vi "_builtins_label_rename.vi"(8 "error in (no error)":errorcluster, 10 "Label":string, 11 "GObject in":refnum<vi>) -> (0 "error out":errorcluster, 2 "has label?":bool, 3 "GObject out":refnum<vi>)   [LabVIEW 2019, in "Script.lvlib"]
doc: "Renames the GObject label if exists and moves the label to the appropriate position.\n\nCreated by: Ryan Pacini"
uses:
  Script.lvlib
  _builtins_label_position.ctl
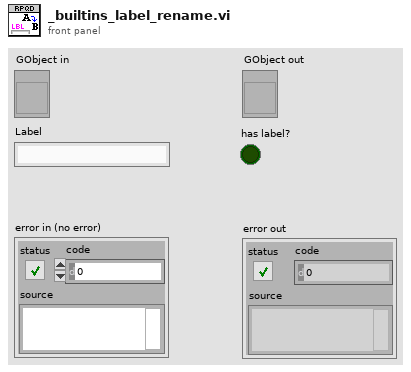
[diagram p1: front panel]
types:
  T1 = typedef "Script.lvlib/_builtins_label_position.ctl" = enum8{"Unchanged", "Top-left", "Top-middle", "Top-right", "Right-top", "Right-middle", "Right-bottom", "Bottom-right", "Bottom-middle", "Bottom-left", "Left-bottom", "Left-middle", "Left-top"}
  T2 = typedef "LVRectTypeDef.ctl" = cluster{"Left":i16, "Top":i16, "Right":i16, "Bottom":i16}
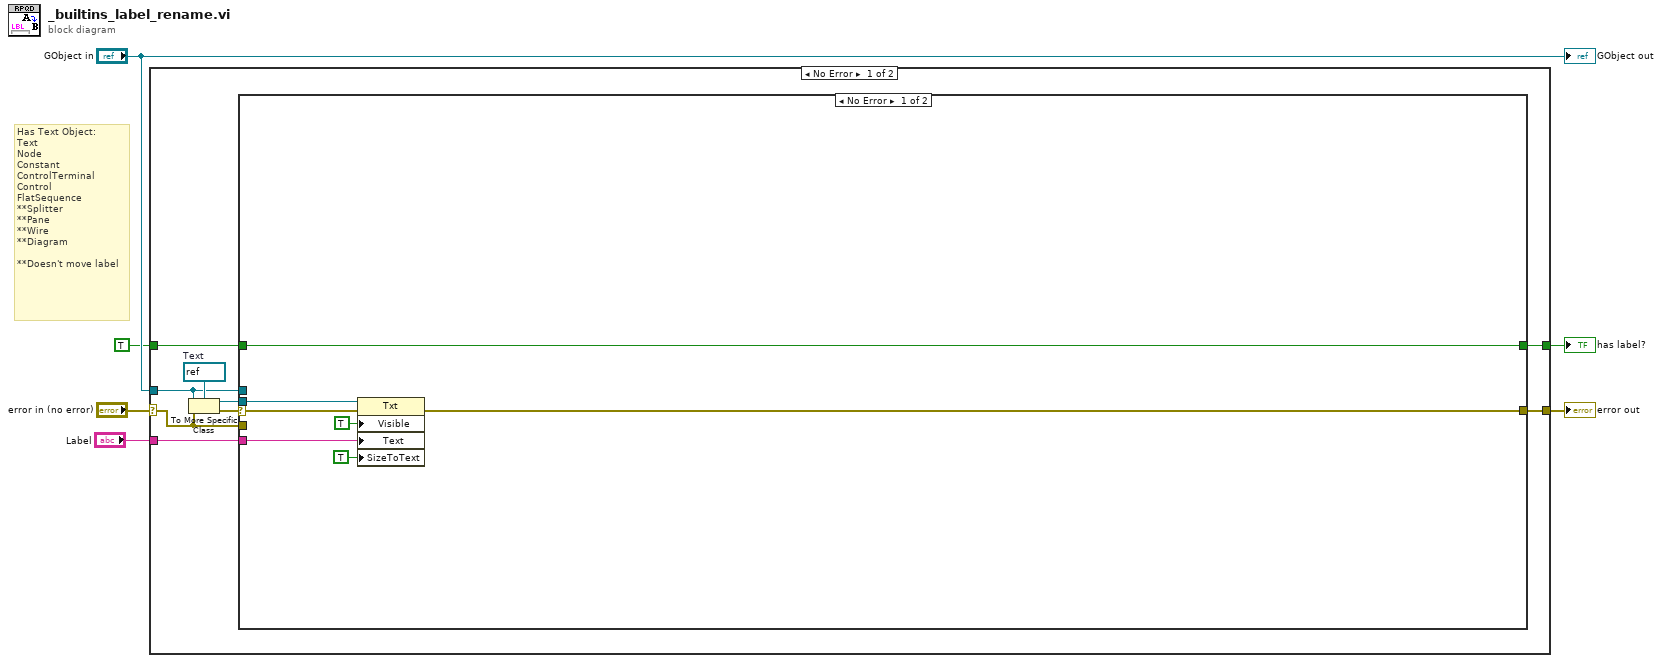
[diagram p0: block diagram]
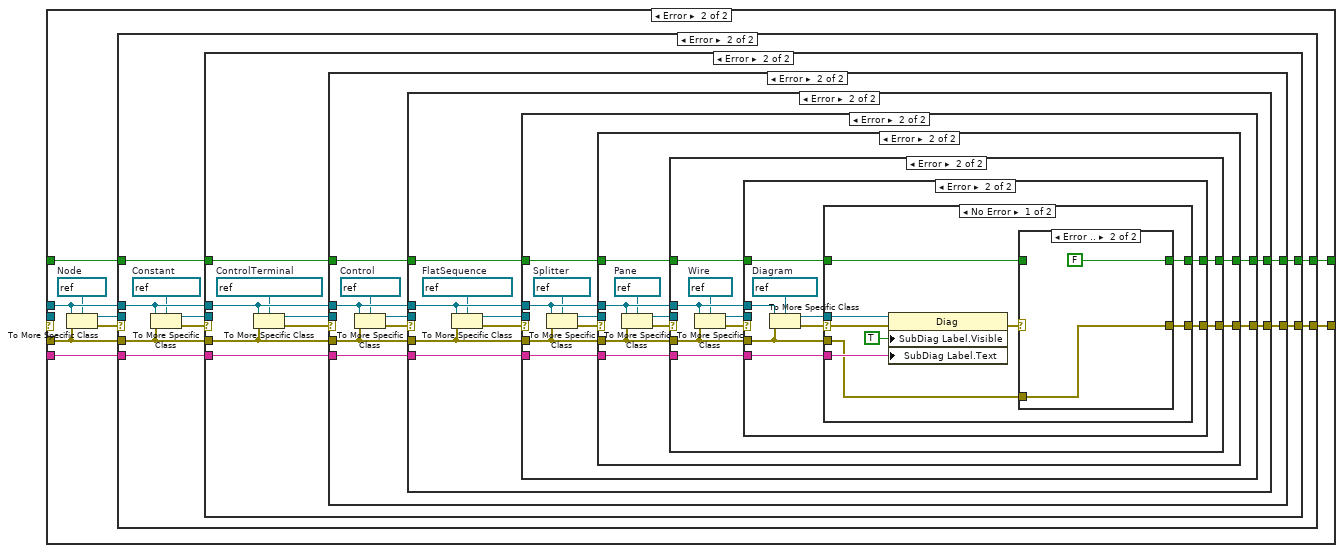
[diagram p2: hidden frame]
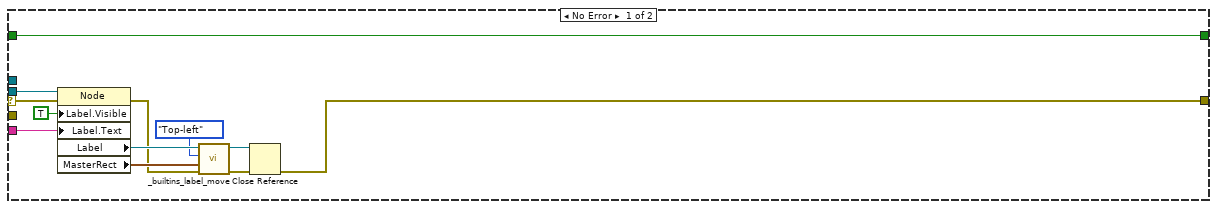
[diagram p3: hidden frame]
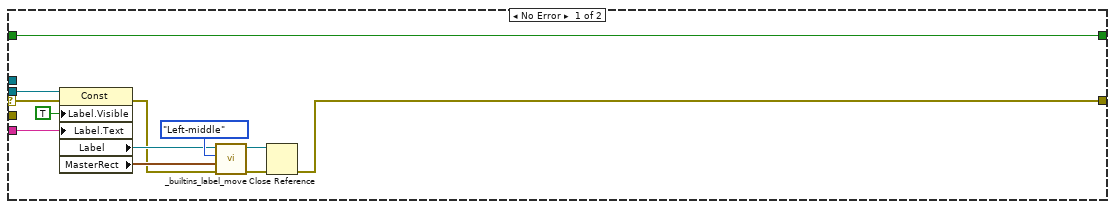
[diagram p4: hidden frame]
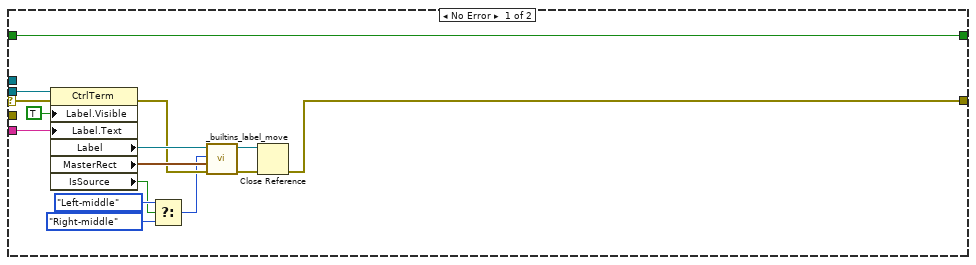
[diagram p5: hidden frame]
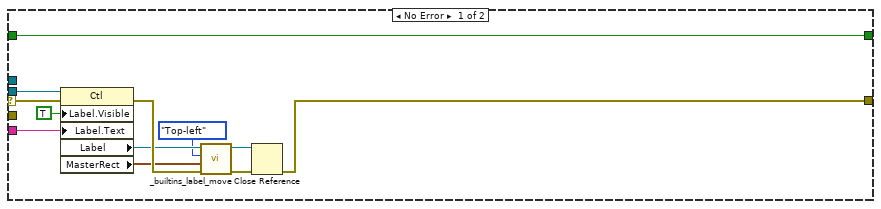
[diagram p6: hidden frame]
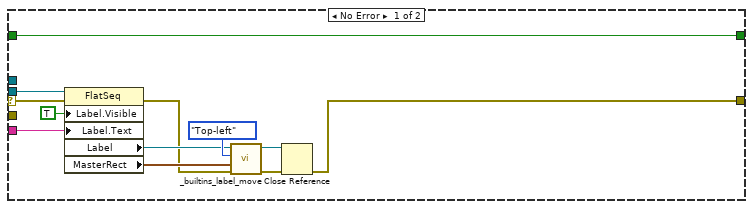
[diagram p7: hidden frame]
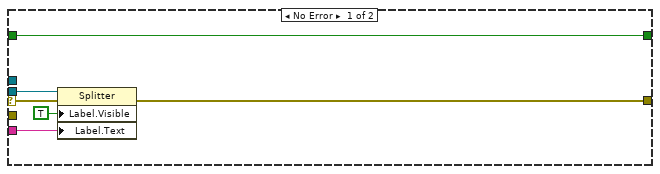
[diagram p8: hidden frame]
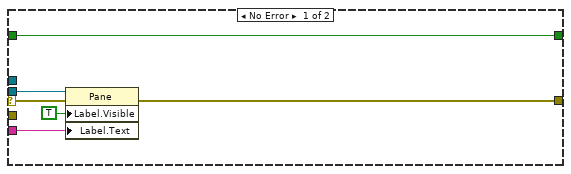
[diagram p9: hidden frame]
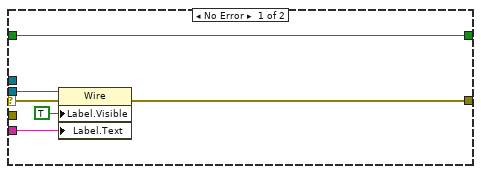
[diagram p10: hidden frame]
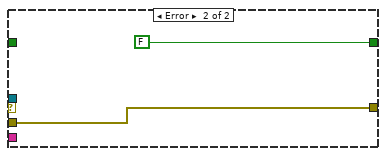
[diagram p12: hidden frame]
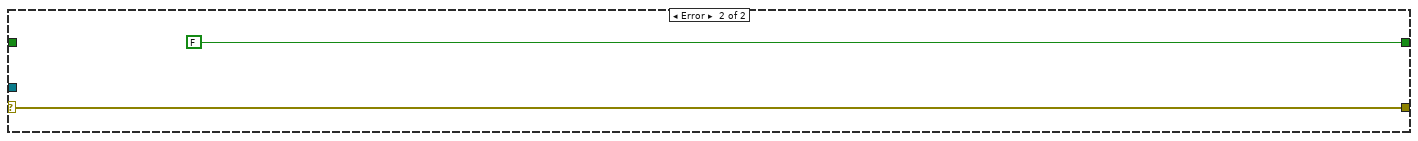
[diagram p13: hidden frame]
diagram:
  # "Has Text Object:\nText\nNode\nConstant\nControlTerminal\nControl\nFlatSequence\n**Splitter\n**Pane\n**Wire\n**Diagram\n\n**Doesn't move label"
  n1 = case shown="No Error" "error in (no error)" {
    selector: "error in (no error)" -> [w10 w201]
    tunnel: "GObject in" -> [w9 _]
    tunnel: [w15 w201] -> w2
    tunnel: [w14 FALSE] -> w3
    tunnel: "Label" -> [w13 _]
    tunnel: TRUE -> [w12 _]
    frame No Error {
      w11 = refnum<vi> refnum  # Text
      n2 = To More Specific Class(target class=w11, reference=w9, error in=w10) -> (specific class reference=w7:refnum<vi>, error out=w8:errorcluster)
      n3 = case shown="No Error" w8 {
        selector: w8 -> [w21 _]
        tunnel: [w18 w31] -> w15
        tunnel: [w17 w30] -> w14
        tunnel: w10 -> [_ w27]
        tunnel: w9 -> [_ w26]
        tunnel: w13 -> [w20 w24]
        tunnel: w12 -> [w17 w23]
        tunnel: w7 -> [w22 _]
        frame No Error {
          n4 = property class="Txt"(reference=w22, error in=w21, "Visible"=TRUE, "Text"=w20, "SizeToText"=TRUE ("Size to Text?")) -> (error out=w18:errorcluster)  [unwired: 1 out]
        }
        frame Error {
          w25 = refnum<vi> refnum  # Node
          n5 = To More Specific Class(target class=w25, reference=w26, error in=w27) -> (specific class reference=w28:refnum<vi>, error out=w29:errorcluster)
          n6 = case shown="Error" w29 {
            selector: w29 -> [w43 _]
            tunnel: w26 -> [_ w50]
            tunnel: w28 -> [w42 _]
            tunnel: w27 -> [_ w49]
            tunnel: [w39 w48] -> w30
            tunnel: [w32 w47] -> w31
            tunnel: w24 -> [w40 w45]
            tunnel: w23 -> [w39 w44]
            frame No Error {
              n7 = property class="Node"(reference=w42, error in=w43, "Label.Visible"=TRUE, "Label.Text"=w40) -> (error out=w33:errorcluster, "Label"=w38:refnum<vi>, "MasterRect"=w37:T2)  [unwired: 1 out]
              n8 = call "_builtins_label_move.vi"("error in (no error)"=w33, "Owner Master Bounds Rect"=w37, "Label Position"=_builtins_label_position."Top-left", "Label in"=w38) -> ("error out"=w36:errorcluster, "dup Label"=w35:refnum<vi>)  [unwired: 6 in]
              n9 = Close Reference(reference=w35, error in (no error)=w36) -> (error out=w32:errorcluster)
            }
            frame Error {
              w46 = refnum<vi> refnum  # Constant
              n10 = To More Specific Class(target class=w46, reference=w50, error in=w49) -> (specific class reference=w51:refnum<vi>, error out=w52:errorcluster)
              n11 = case shown="Error" w52 {
                selector: w52 -> [w64 _]
                tunnel: w51 -> [w63 _]
                tunnel: w50 -> [_ w71]
                tunnel: w49 -> [_ w70]
                tunnel: [w60 w68] -> w48
                tunnel: [w53 w69] -> w47
                tunnel: w45 -> [w62 w66]
                tunnel: w44 -> [w60 w65]
                frame No Error {
                  n12 = property class="Const"(reference=w63, error in=w64, "Label.Visible"=TRUE, "Label.Text"=w62) -> (error out=w54:errorcluster, "Label"=w56:refnum<vi>, "MasterRect"=w55:T2)  [unwired: 1 out]
                  n13 = call "_builtins_label_move.vi"("error in (no error)"=w54, "Owner Master Bounds Rect"=w55, "Label Position"=_builtins_label_position."Left-middle", "Label in"=w56) -> ("error out"=w59:errorcluster, "dup Label"=w58:refnum<vi>)  [unwired: 6 in]
                  n14 = Close Reference(reference=w58, error in (no error)=w59) -> (error out=w53:errorcluster)
                }
                frame Error {
                  w67 = refnum<vi> refnum  # ControlTerminal
                  n15 = To More Specific Class(target class=w67, reference=w71, error in=w70) -> (specific class reference=w72:refnum<vi>, error out=w73:errorcluster)
                  n16 = case shown="Error" w73 {
                    selector: w73 -> [w88 _]
                    tunnel: w72 -> [w87 _]
                    tunnel: w71 -> [_ w95]
                    tunnel: w70 -> [_ w94]
                    tunnel: [w78 w93] -> w69
                    tunnel: [w84 w92] -> w68
                    tunnel: w66 -> [w86 w90]
                    tunnel: w65 -> [w84 w89]
                    frame No Error {
                      n17 = property class="CtrlTerm"(reference=w87, error in=w88, "Label.Visible"=TRUE, "Label.Text"=w86) -> (error out=w79:errorcluster, "Label"=w81:refnum<vi>, "MasterRect"=w80:T2, "IsSource"=w75:bool)  [unwired: 1 out]
                      n18 = Select(t=_builtins_label_position."Left-middle" ("Label Position"), s=w75, f=_builtins_label_position."Right-middle" ("Label Position")) -> (s? t:f=w74:T1)
                      n19 = call "_builtins_label_move.vi"("error in (no error)"=w79, "Owner Master Bounds Rect"=w80, "Label Position"=w74, "Label in"=w81) -> ("error out"=w83:errorcluster, "dup Label"=w82:refnum<vi>)  [unwired: 6 in]
                      n20 = Close Reference(reference=w82, error in (no error)=w83) -> (error out=w78:errorcluster)
                    }
                    frame Error {
                      w91 = refnum<vi> refnum  # Control
                      n21 = To More Specific Class(target class=w91, reference=w95, error in=w94) -> (specific class reference=w96:refnum<vi>, error out=w97:errorcluster)
                      n22 = case shown="Error" w97 {
                        selector: w97 -> [w109 _]
                        tunnel: w96 -> [w108 _]
                        tunnel: w95 -> [_ w113]
                        tunnel: w94 -> [_ w116]
                        tunnel: [w101 w114] -> w93
                        tunnel: [w105 w115] -> w92
                        tunnel: w90 -> [w107 w111]
                        tunnel: w89 -> [w105 w110]
                        frame No Error {
                          n23 = property class="Ctl"(reference=w108, error in=w109, "Label.Visible"=TRUE, "Label.Text"=w107) -> (error out=w102:errorcluster, "Label"=w100:refnum<vi>, "MasterRect"=w99:T2)  [unwired: 1 out]
                          n24 = call "_builtins_label_move.vi"("error in (no error)"=w102, "Owner Master Bounds Rect"=w99, "Label Position"=_builtins_label_position."Top-left", "Label in"=w100) -> ("error out"=w104:errorcluster, "dup Label"=w103:refnum<vi>)  [unwired: 6 in]
                          n25 = Close Reference(reference=w103, error in (no error)=w104) -> (error out=w101:errorcluster)
                        }
                        frame Error {
                          w112 = refnum<vi> refnum  # FlatSequence
                          n26 = To More Specific Class(target class=w112, reference=w113, error in=w116) -> (specific class reference=w117:refnum<vi>, error out=w118:errorcluster)
                          n27 = case shown="Error" w118 {
                            selector: w118 -> [w130 _]
                            tunnel: w117 -> [w129 _]
                            tunnel: w116 -> [_ w137]
                            tunnel: [w126 w134] -> w115
                            tunnel: [w119 w135] -> w114
                            tunnel: w113 -> [_ w138]
                            tunnel: w111 -> [w128 w132]
                            tunnel: w110 -> [w126 w131]
                            frame No Error {
                              n28 = property class="FlatSeq"(reference=w129, error in=w130, "Label.Visible"=TRUE, "Label.Text"=w128) -> (error out=w120:errorcluster, "Label"=w122:refnum<vi>, "MasterRect"=w121:T2)  [unwired: 1 out]
                              n29 = call "_builtins_label_move.vi"("error in (no error)"=w120, "Owner Master Bounds Rect"=w121, "Label Position"=_builtins_label_position."Top-left", "Label in"=w122) -> ("error out"=w125:errorcluster, "dup Label"=w124:refnum<vi>)  [unwired: 6 in]
                              n30 = Close Reference(reference=w124, error in (no error)=w125) -> (error out=w119:errorcluster)
                            }
                            frame Error {
                              w133 = refnum<vi> refnum  # Splitter
                              n31 = To More Specific Class(target class=w133, reference=w138, error in=w137) -> (specific class reference=w136:refnum<vi>, error out=w139:errorcluster)
                              n32 = case shown="Error" w139 {
                                selector: w139 -> [w144 _]
                                tunnel: w138 -> [_ w149]
                                tunnel: w137 -> [_ w153]
                                tunnel: w136 -> [w145 _]
                                tunnel: [w140 w152] -> w135
                                tunnel: [w141 w151] -> w134
                                tunnel: w132 -> [w143 w147]
                                tunnel: w131 -> [w141 w146]
                                frame No Error {
                                n33 = property class="Splitter"(reference=w145, error in=w144, "Label.Visible"=TRUE, "Label.Text"=w143) -> (error out=w140:errorcluster)  [unwired: 1 out]
                                }
                                frame Error {
                                w148 = refnum<vi> refnum  # Pane
                                n34 = To More Specific Class(target class=w148, reference=w149, error in=w153) -> (specific class reference=w150:refnum<vi>, error out=w154:errorcluster)
                                n35 = case shown="Error" w154 {
                                selector: w154 -> [w160 _]
                                tunnel: w153 -> [_ w166]
                                tunnel: [w155 w165] -> w152
                                tunnel: [w156 w169] -> w151
                                tunnel: w150 -> [w159 _]
                                tunnel: w149 -> [_ w164]
                                tunnel: w147 -> [w157 w162]
                                tunnel: w146 -> [w156 w161]
                                frame No Error {
                                n36 = property class="Pane"(reference=w159, error in=w160, "Label.Visible"=TRUE, "Label.Text"=w157) -> (error out=w155:errorcluster)  [unwired: 1 out]
                                }
                                frame Error {
                                w163 = refnum<vi> refnum  # Wire
                                n37 = To More Specific Class(target class=w163, reference=w164, error in=w166) -> (specific class reference=w167:refnum<vi>, error out=w168:errorcluster)
                                n38 = case shown="Error" w168 {
                                selector: w168 -> [w174 _]
                                tunnel: [w171 w184] -> w169
                                tunnel: w167 -> [w175 _]
                                tunnel: w166 -> [_ w180]
                                tunnel: [w170 w179] -> w165
                                tunnel: w164 -> [_ w183]
                                tunnel: w162 -> [w173 w177]
                                tunnel: w161 -> [w171 w176]
                                frame No Error {
                                n39 = property class="Wire"(reference=w175, error in=w174, "Label.Visible"=TRUE, "Label.Text"=w173) -> (error out=w170:errorcluster)  [unwired: 1 out]
                                }
                                frame Error {
                                w178 = refnum<vi> refnum  # Diagram
                                n40 = To More Specific Class(target class=w178, reference=w183, error in=w180) -> (specific class reference=w181:refnum<vi>, error out=w182:errorcluster)
                                n41 = case shown="No Error" w182 {
                                selector: w182 -> [w189 _]
                                tunnel: [w190 FALSE] -> w184
                                tunnel: w181 -> [w193 _]
                                tunnel: w180 -> [w187 w198]
                                tunnel: [w191 w198] -> w179
                                tunnel: w177 -> [w188 _]
                                tunnel: w176 -> [w186 _]
                                frame No Error {
                                n42 = property class="Diag"(reference=w193, error in=w189, "SubDiag Label.Visible"=TRUE ("Subdiagram Label.Visible"), "SubDiag Label.Text"=w188) -> (error out=w192:errorcluster)  [unwired: 1 out]
                                n43 = case shown="Error .." w192 {
                                selector: w192 -> [w195 _]
                                tunnel: [w195 w197] -> w191
                                tunnel: [w194 FALSE] -> w190
                                tunnel: w187 -> [_ w197]
                                tunnel: w186 -> [w194 _]
                                frame No Error {
                                }
                                frame Error {
                                }
                                }
                                }
                                frame Error {
                                }
                                }
                                }
                                }
                                }
                                }
                                }
                              }
                            }
                          }
                        }
                      }
                    }
                  }
                }
              }
            }
          }
        }
      }
    }
    frame Error {
    }
  }
  "error out" <- w2
  "has label?" <- w3
  "GObject out" <- "GObject in"
